vi "New Object Name Dialog.vi"(8 "error in (no error)":errorcluster, 9 "String Name (\"object\")":string="object", 10 "Object Name in":string, 11 "Enable":bool=TRUE) -> (0 "error out":errorcluster, 1 "OK":bool, 2 "Object Name out":string)   [LabVIEW 2019]
doc: "Displays a standard dialog box that prompts users to enter information, such as a user name and password.\n--------------------\n\nThis Express VI is configured as follows:\n\nMessage to Display to the User:Enter a name for the new ROI:\nThe inputs are: \nText Entry Box: ROI Name"
panel:
  in  "Object Name":string caption="ROI Name"
  out "String":string="Enter a name for the ROI:"
  in  "Cancel":bool
  in  "OK1":bool
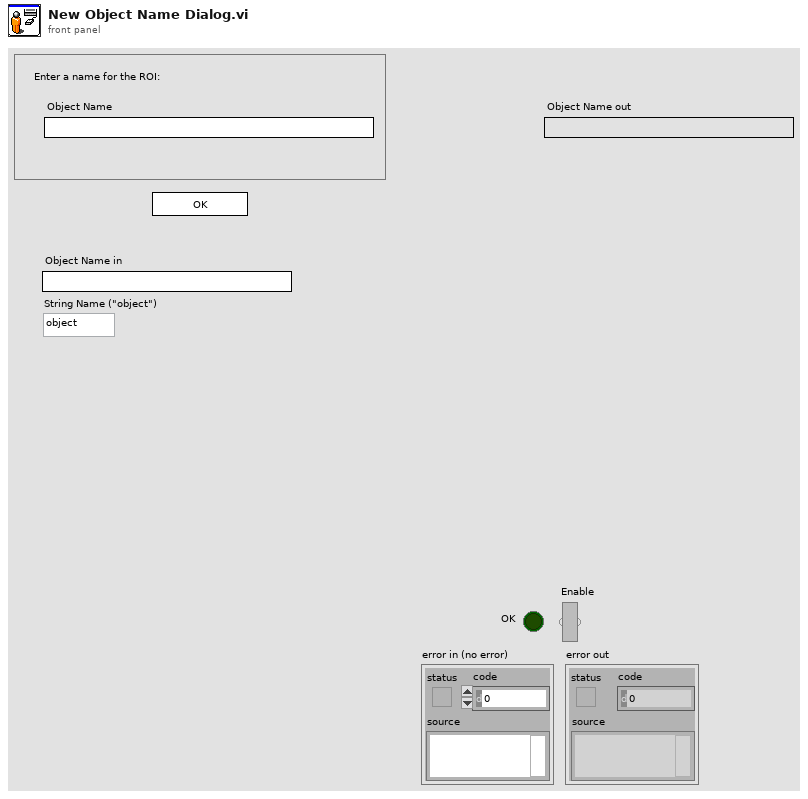
[diagram p1: front panel]
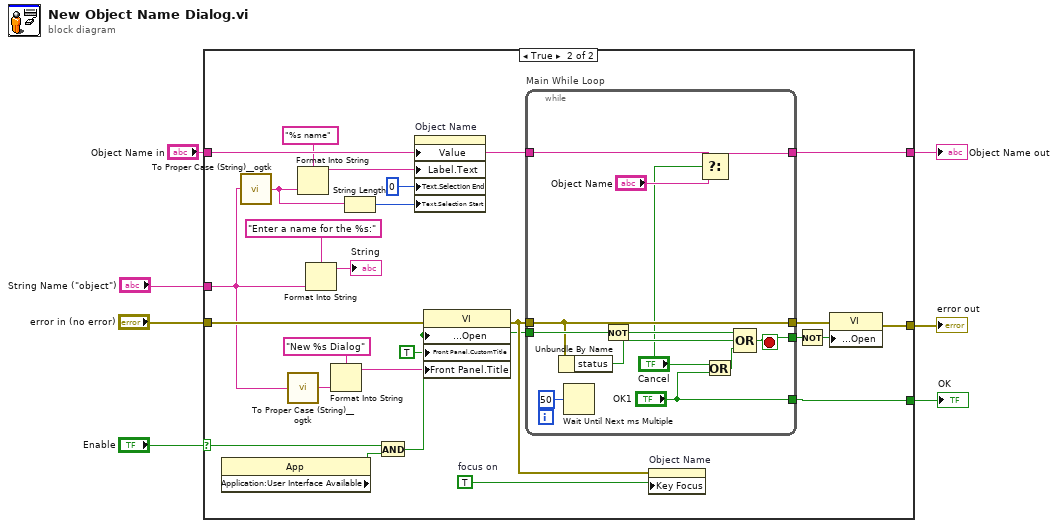
[diagram p0: block diagram]
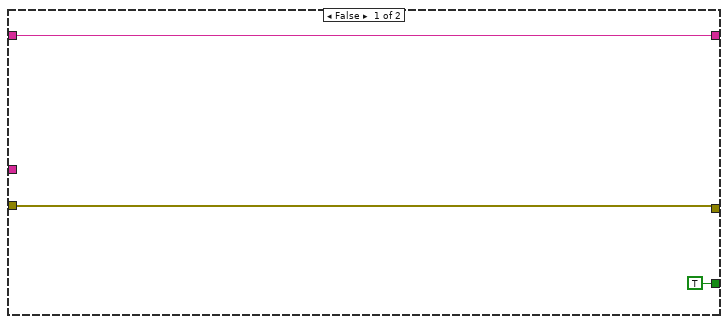
[diagram p2: hidden frame]
diagram:
  n1 = case shown="True" "Enable" {
    selector: "Enable" -> [_ w28]
    tunnel: [TRUE ("OK1") w35] -> w7
    tunnel: "error in (no error)" -> [w9 w31]
    tunnel: [w9 w29] -> w5
    tunnel: [w10 w25] -> w3
    tunnel: "Object Name in" -> [w10 w21]
    tunnel: "String Name (\"object\")" -> [_ w15]
    frame False {
    }
    frame True {
      w24 = TRUE  # focus on
      n2 = property class="App"() -> ("Application:User Interface Available"=w26:bool)  [unwired: 2 in, 2 out]
      n3 = call <userlib>:"To Proper Case (String)__ogtk.vi"("string"=w15) -> ("proper case string"=w12:string)  [unwired: 4 in]
      n4 = call <userlib>:"To Proper Case (String)__ogtk.vi"("string"=w15) -> ("proper case string"=w16:string)  [unwired: 4 in]
      n5 = Format Into String(format string="%s name", w12) -> (resulting string=w20:string)  [unwired: 2 in, 1 out]
      n6 = Format Into String(format string="Enter a name for the %s:" ("String"), w15) -> (resulting string=→"String":string)  [unwired: 2 in, 1 out]
      n7 = Format Into String(format string="New %s Dialog", w16) -> (resulting string=w14:string)  [unwired: 2 in, 1 out]
      n8 = String Length(string=w12) -> (length=w11:i32)
      n9 = And(x=w28, y=w26) -> (x .and. y?=w27:bool)
      n10 = property on="Object Name" class="Str"("Value"=w21, "Label.Text"=w20, "Text.Selection End"=u32 0 ("Text.Selection:End"), "Text.Selection Start"=w11) -> ()  [unwired: 2 in, 2 out]
      n11 = property class="VI"(error in=w31, "Front Panel Window:Open"=w27, "Front Panel.CustomTitle"=TRUE ("Front Panel Window:Custom Title"), "Front Panel.Title"=w14) -> (error out=w32:errorcluster)  [unwired: 1 in, 1 out]
      n12 = while "Main While Loop" {
        tunnel: ["OK1"] -> w35
        tunnel: w27 -> [w45]
        tunnel: [w43] -> w33
        tunnel: w32 -> [w42]
        tunnel: [w42] -> w30
        tunnel: [w38] -> w25
        tunnel: w21 -> [w36]
        stop <- w43 stop-if-true
        n13 = Unbundle By Name(w42) -> ("status"=w40:bool)
        n14 = Wait Until Next ms Multiple(millisecond multiple=u32 50) -> ()  [unwired: 1 out]
        n15 = Not(x=w45) -> (.not. x?=w44:bool)
        n16 = Select(t=w36, s="Cancel", f="Object Name") -> (s? t:f=w38:string)
        n17 = Or(x="Cancel", y="OK1") -> (x .or. y?=w41:bool)
        n18 = Compound Arithmetic op=OR(w44, w40, w41) -> (w43:bool)
      }
      n19 = property on="Object Name" class="Str"(error in=w32, "Key Focus"=w24) -> ()  [unwired: 1 in, 2 out]
      n20 = Not(x=w33) -> (.not. x?=w34:bool)
      n21 = property class="VI"(error in=w30, "Front Panel Window:Open"=w34) -> (error out=w29:errorcluster)  [unwired: 1 in, 1 out]
    }
  }
  "OK" <- w7
  "error out" <- w5
  "Object Name out" <- w3
